vi "SR830 lock to phase tw.vi"(7 "Osc. Freq. (Hz)":dbl=1126.0 min=0.001 max=250000.0 step=0.001 format="%.3f", 8 "Lock in parameters":T1={"Phase (deg)"=82.0, "TC"=7, "TC Multiplier"=5.0} {"TC Multiplier" min=0.0 max=10.0 step=1.0 format="%.2f"; "TC" items=["10 µs", "30 µs", "100 µs", "300 µs", "1 ms", "3 ms", "10 ms", "30 ms", "100 ms", "300 ms", "1 s", "3 s", "10 s", "30 s", "100 s", "300 s", "1 ks", "3 ks", "10 ks", "30 ks"]; "Phase (deg)" format="%.3f"}, 9 "Lock-in GPIB address":string="0:9", 10 "SRS DS345 GPIB address":string="0:19") -> ()   [LabVIEW 2015]
uses:
  Global vab.vi
panel:
  in  "Lock-in GPIB address  (Fake)":string="1:8"
  out "Signal (A)":dbl format="%#_6p"
  out "step time (ms)":u32=102
  out "Waveform Chart":dbl(graph)
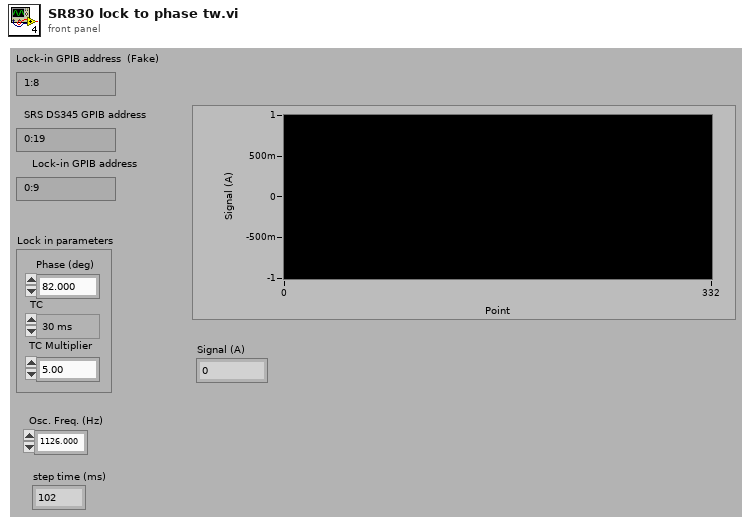
[diagram p1: front panel]
types:
  T1 = cluster{"Phase (deg)":dbl, "TC":i32, "TC Multiplier":dbl}
  T2 = cluster{"Lock-in GPIB address  (Fake)":string, "Lock-in GPIB address  ":string, "SRS DS345 GPIB address":string}
  T3 = cluster{"f,x1,y1,x2,y2,aux11,aux12[0]":dbl, "f,x1,y1,x2,y2,aux11,aux12[1]":dbl, "f,x1,y1,x2,y2,aux11,aux12[2]":dbl, "f,x1,y1,x2,y2,aux11,aux12[3]":dbl, "f,x1,y1,x2,y2,aux11,aux12[4]":dbl, "f,x1,y1,x2,y2,aux11,aux12[5]":dbl, "f,x1,y1,x2,y2,aux11,aux12[6]":dbl}
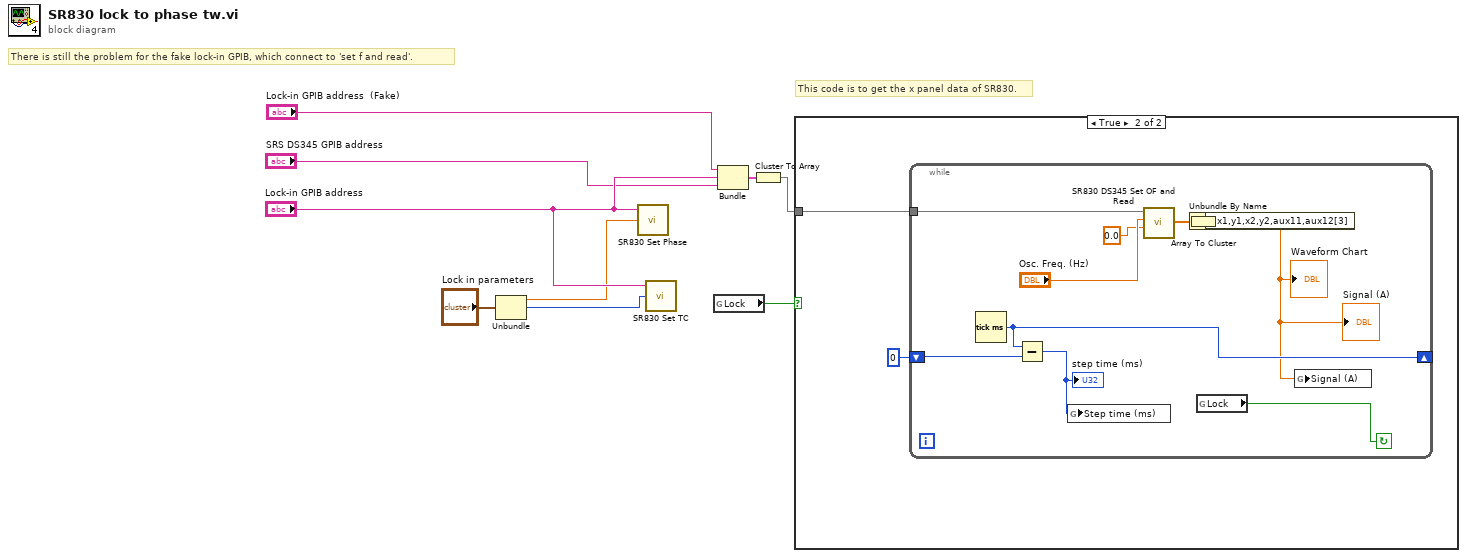
[diagram p0: block diagram]
diagram:
  # "This code is to get the x panel data of SR830."
  # "There is still the problem for the fake lock-in GPIB, which connect to 'set f and read'."
  n1 = Unbundle("Lock in parameters") -> ("Phase (deg)"=w3:dbl, "TC"=w2:i32)  [unwired: 1 out]
  n2 = call "SR830 Set Phase.vi"("Phase (deg)"=w3, "GPIB address"="Lock-in GPIB address") -> ()  [unwired: 2 in, 2 out]
  n3 = call "SR830 Set TC.vi"("time constant\n(10 µs : 0)"=w2, "GPIB address"="Lock-in GPIB address") -> ()  [unwired: 1 in, 3 out]
  n4 = global read "Global vab.vi" "Lock"() -> (w1:bool)
  n5 = Bundle("Lock-in GPIB address  (Fake)"="Lock-in GPIB address  (Fake)", "Lock-in GPIB address"="Lock-in GPIB address", "SRS DS345 GPIB address"="SRS DS345 GPIB address") -> (w6:T2)  [unwired: 1 out]
  n6 = Cluster To Array(cluster=w6) -> (array=w5:string[])
  n7 = case shown="True" w1 {
    tunnel: w5 -> [_ w10]
    frame False {
    }
    frame True {
      n8 = while {
        shift-right: [w20] -> _
        shift-left: 0 -> [w21]
        tunnel: w10 -> [w15]
        stop <- w12 continue-if-true
        n9 = Tick Count (ms)() -> (millisecond timer value=w20:u32)
        n10 = Subtract(x=w20, y=w21) -> (x-y=w14:u32)
        "step time (ms)" <- w14
        n11 = global write "Global vab.vi" "Step time (ms)"(w14) -> ()
        n12 = call "SR830 DS345 Set OF and Read.vi"("Wait Time (sec)"=0.0, "Oscillator Frequency (Hz)"="Osc. Freq. (Hz)", "GPIB addresses"=w15) -> ("f,x1,y1,x2,y2,aux11,aux12"=w18:dbl[])  [unwired: 1 in, 1 out]
        n13 = Array To Cluster(array=w18) -> (cluster=w19:T3)
        n14 = Unbundle By Name(w19) -> ("f,x1,y1,x2,y2,aux11,aux12[3]"=w13:dbl)
        "Waveform Chart" <- w13
        "Signal (A)" <- w13
        n15 = global read "Global vab.vi" "Lock"() -> (w12:bool)
        n16 = global write "Global vab.vi" "Signal (A)"(w13) -> ()
      }
    }
  }
